vi "main_VI.vi"() -> ()   [LabVIEW 2011]
doc: "This example VI shows how to use thermocouples to take a temperature measurement.\n\nNote:\nFor front panel measurements, make sure the Input switch is in the out position(F)\nFor plug-in card measurements, make sure the Input switch is in the in poisition(R)"
uses:
  <instrlib>/Keithley 622x LV 2009/Configure/Source/Typedefs/KE622x -- Current Level.ctl
  <instrlib>/Keithley 622x LV 2009/Typedefs/KE622x -- On Off Control.ctl
  <vilib>/Utility/file.llb/Write To Spreadsheet File (string).vi
  sub_VIs/west_controller/p6100_write.vi
  <vilib>/addons/Fuzzy Logic/FL Fuzzy Controller (MISO).vi
  <instrlib>/Keithley 27XX/Public/Data/Read Multiple Direct.vi
  sub_VIs/west_controller/p6100_write_setpoint.vi
  <instrlib>/Keithley 27XX/Keithley 27XX.lvlib
  <instrlib>/Keithley 622x LV 2009/Keithley 622x.lvlib
  <vilib>/addons/Fuzzy Logic/NI_Fuzzy_Logic_API.lvlib
panel:
  in  "Current Level (A) In":T1=0.1 min=-0.105 max=0.105 format="%.4p"
  out "Seebeck Graph":cluster{"Y":dbl[], "Y":dbl[]}[](graph)=[{"Y"=[29.390292420231198], "Y"=[134.49214421747814]}]
  out "Resistivity Graph":cluster{"Y":dbl[], "Y":dbl[]}[](graph)=[{"Y"=[29.33802939652643], "Y"=[inf]}]
  out "Temp Graph":cluster{"Y":dbl[], "Y":dbl[]}[](graph)=[{"Y"=[0.0, 0.0, 0.0, 0.0, 0.0, 0.0, 0.0, 0.0, 0.0, 0.0, 0.0, 0.0, 0.0, 0.0, 0.0, 0.0, 0.0, 0.0, 0.0, 0.0, 0.0, 0.0, 0.0, 0.0, 0.0, 0.0, 0.0, 0.0, 0.0, 0.0, 0.0, 0.0, 0.0, 0.0, 0.0, 0.0, 0.0, 0.0, 0.0, 0.0, 0.0, 0.0, 0.0, 0.0, 0.0, 0.0, 0.0, 0.0, 0.0, 0.0, 0.0, 0.0, 0.0, 0.0, 0.0, 0.0, 0.0, 0.0, 0.0, 0.0, 0.0, 0.0, 0.0, 0.0, 0.0, 0.0, 0.0, 0.0, 0.0, 0.0, 0.0, 0.0, 0.0, 0.0, 0.0, 0.0, 0.0, 0.0, 0.0, 0.0, 0.0, 0.0, 0.0, 0.0, 0.0, 0.0, 0.0, 0.0, 0.0, 0.0, 0.0, 0.0, 0.0, 0.0, 0.0, 0.0, 0.0, 0.0, 0.0, 0.0], "Y"=[22.79692727272725, 0.0, 0.0, 0.0, 0.0, 0.0, 0.0, 0.0, 0.0, 0.0, 0.0, 0.0, 0.0, 0.0, 0.0, 0.0, 0.0, 0.0, 0.0, 0.0, 0.0, 0.0, 0.0, 0.0, 0.0, 0.0, 0.0, 0.0, 0.0, 0.0, 0.0, 0.0, 0.0, 0.0, 0.0, 0.0, 0.0, 0.0, 0.0, 0.0, 0.0, 0.0, 0.0, 0.0, 0.0, 0.0, 0.0, 0.0, 0.0, 0.0, 0.0, 0.0, 0.0, 0.0, 0.0, 0.0, 0.0, 0.0, 0.0, 0.0, 0.0, 0.0, 0.0, 0.0, 0.0, 0.0, 0.0, 0.0, 0.0, 0.0, 0.0, 0.0, 0.0, 0.0, 0.0, 0.0, 0.0, 0.0, 0.0, 0.0, 0.0, 0.0, 0.0, 0.0, 0.0, 0.0, 0.0, 0.0, 0.0, 0.0, 0.0, 0.0, 0.0, 0.0, 0.0, 0.0, 0.0, 0.0, 0.0, 0.0]}, {"Y"=[0.0, 0.0, 0.0, 0.0, 0.0, 0.0, 0.0, 0.0, 0.0, 0.0, 0.0, 0.0, 0.0, 0.0, 0.0, 0.0, 0.0, 0.0, 0.0, 0.0, 0.0, 0.0, 0.0, 0.0, 0.0, 0.0, 0.0, 0.0, 0.0, 0.0, 0.0, 0.0, 0.0, 0.0, 0.0, 0.0, 0.0, 0.0, 0.0, 0.0, 0.0, 0.0, 0.0, 0.0, 0.0, 0.0, 0.0, 0.0, 0.0, 0.0, 0.0, 0.0, 0.0, 0.0, 0.0, 0.0, 0.0, 0.0, 0.0, 0.0, 0.0, 0.0, 0.0, 0.0, 0.0, 0.0, 0.0, 0.0, 0.0, 0.0, 0.0, 0.0, 0.0, 0.0, 0.0, 0.0, 0.0, 0.0, 0.0, 0.0, 0.0, 0.0, 0.0, 0.0, 0.0, 0.0, 0.0, 0.0, 0.0, 0.0, 0.0, 0.0, 0.0, 0.0, 0.0, 0.0, 0.0, 0.0, 0.0, 0.0], "Y"=[29.252771602137226, 0.0, 0.0, 0.0, 0.0, 0.0, 0.0, 0.0, 0.0, 0.0, 0.0, 0.0, 0.0, 0.0, 0.0, 0.0, 0.0, 0.0, 0.0, 0.0, 0.0, 0.0, 0.0, 0.0, 0.0, 0.0, 0.0, 0.0, 0.0, 0.0, 0.0, 0.0, 0.0, 0.0, 0.0, 0.0, 0.0, 0.0, 0.0, 0.0, 0.0, 0.0, 0.0, 0.0, 0.0, 0.0, 0.0, 0.0, 0.0, 0.0, 0.0, 0.0, 0.0, 0.0, 0.0, 0.0, 0.0, 0.0, 0.0, 0.0, 0.0, 0.0, 0.0, 0.0, 0.0, 0.0, 0.0, 0.0, 0.0, 0.0, 0.0, 0.0, 0.0, 0.0, 0.0, 0.0, 0.0, 0.0, 0.0, 0.0, 0.0, 0.0, 0.0, 0.0, 0.0, 0.0, 0.0, 0.0, 0.0, 0.0, 0.0, 0.0, 0.0, 0.0, 0.0, 0.0, 0.0, 0.0, 0.0, 0.0]}, {"Y"=[0.0, 0.0, 0.0, 0.0, 0.0, 0.0, 0.0, 0.0, 0.0, 0.0, 0.0, 0.0, 0.0, 0.0, 0.0, 0.0, 0.0, 0.0, 0.0, 0.0, 0.0, 0.0, 0.0, 0.0, 0.0, 0.0, 0.0, 0.0, 0.0, 0.0, 0.0, 0.0, 0.0, 0.0, 0.0, 0.0, 0.0, 0.0, 0.0, 0.0, 0.0, 0.0, 0.0, 0.0, 0.0, 0.0, 0.0, 0.0, 0.0, 0.0, 0.0, 0.0, 0.0, 0.0, 0.0, 0.0, 0.0, 0.0, 0.0, 0.0, 0.0, 0.0, 0.0, 0.0, 0.0, 0.0, 0.0, 0.0, 0.0, 0.0, 0.0, 0.0, 0.0, 0.0, 0.0, 0.0, 0.0, 0.0, 0.0, 0.0, 0.0, 0.0, 0.0, 0.0, 0.0, 0.0, 0.0, 0.0, 0.0, 0.0, 0.0, 0.0, 0.0, 0.0, 0.0, 0.0, 0.0, 0.0, 0.0, 0.0], "Y"=[29.52781323832517, 0.0, 0.0, 0.0, 0.0, 0.0, 0.0, 0.0, 0.0, 0.0, 0.0, 0.0, 0.0, 0.0, 0.0, 0.0, 0.0, 0.0, 0.0, 0.0, 0.0, 0.0, 0.0, 0.0, 0.0, 0.0, 0.0, 0.0, 0.0, 0.0, 0.0, 0.0, 0.0, 0.0, 0.0, 0.0, 0.0, 0.0, 0.0, 0.0, 0.0, 0.0, 0.0, 0.0, 0.0, 0.0, 0.0, 0.0, 0.0, 0.0, 0.0, 0.0, 0.0, 0.0, 0.0, 0.0, 0.0, 0.0, 0.0, 0.0, 0.0, 0.0, 0.0, 0.0, 0.0, 0.0, 0.0, 0.0, 0.0, 0.0, 0.0, 0.0, 0.0, 0.0, 0.0, 0.0, 0.0, 0.0, 0.0, 0.0, 0.0, 0.0, 0.0, 0.0, 0.0, 0.0, 0.0, 0.0, 0.0, 0.0, 0.0, 0.0, 0.0, 0.0, 0.0, 0.0, 0.0, 0.0, 0.0, 0.0]}]
  in  "Comments":string="Esto es una prueba"
  in  "play":bool
  in  "stop":bool
  out "Tab Control 2":enum32{"Page 1", "Page 3"}(tab)
  in  "D (mm)":dbl=7.5
  in  "H (mm)":dbl=1.3
  in  "B (mm)":dbl
  in  "A (mm)":dbl
  in  "L (mm)":dbl
  in  "Select type":u16(ring) items=["Cylinder", "Rectangular"]
  in  "file path":path
  in  "SetPoint Top":dbl
  in  "SetPoint Bottom":dbl
  # "SAMPLE TYPE"
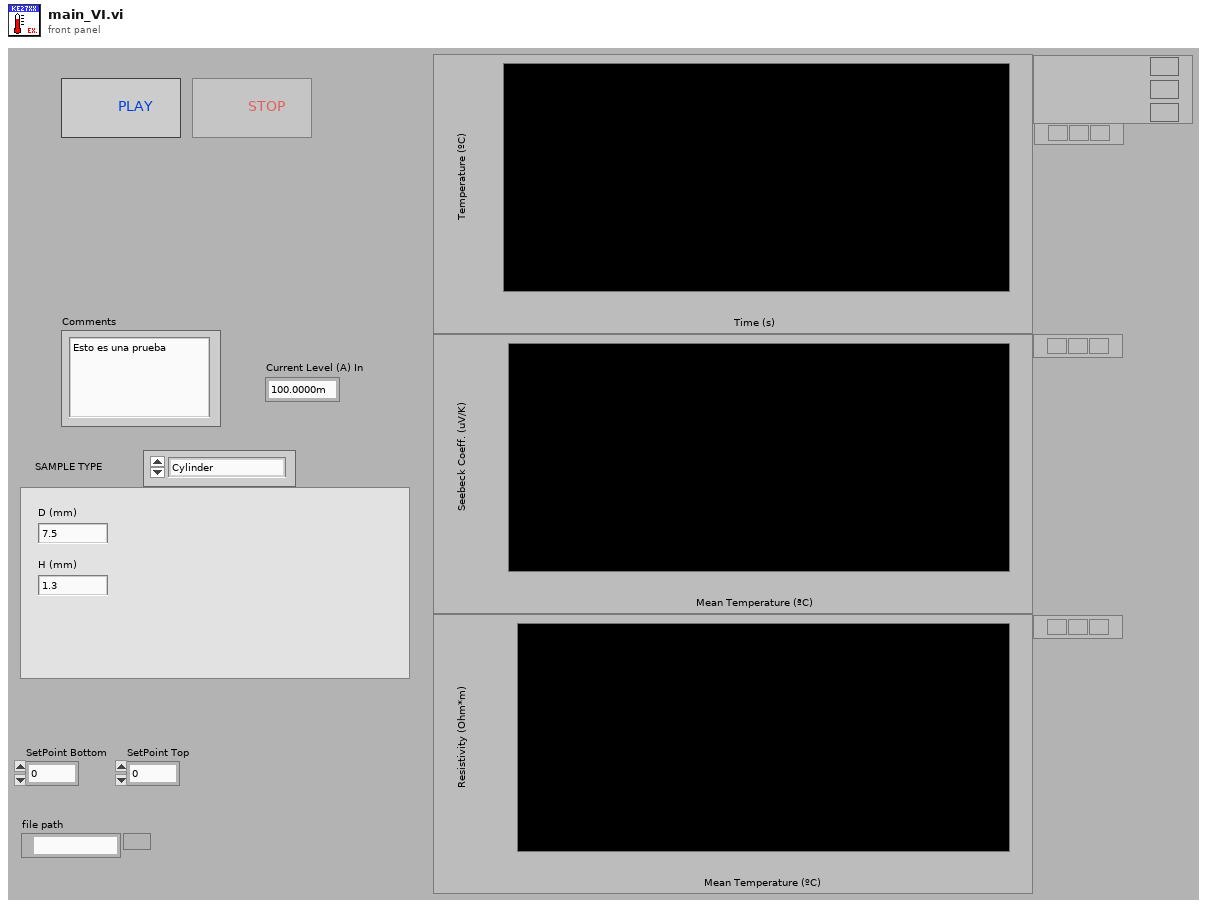
[diagram p1: front panel]
types:
  T1 = typedef "Keithley 622x.lvlib/KE622x -- Current Level.ctl" = dbl
  T2 = cluster{"Baud Rate (9600)":u32, "Flow Control (1: XON/XOFF)":u16, "Termination Char (0:CR)":u16}
  T3 = cluster{"Mode":enum16{"RTU", "ASCII"}, "Slave Bottom":u8, "Slave Top":u8}
  T4 = enum8{"Enabled", "Disabled", "Disabled and Grayed Out"}
  T5 = typedef "NI_Fuzzy_Logic_API.lvlib/FL System.ctl" = cluster{"input variables":T6[], "output variables":T6[], "rules":T9[], "defuzzification method":T15, "description":string, "user MF interpolating polynomials":T16[]}
  T6 = typedef "NI_Fuzzy_Logic_API.lvlib/FL Variable.ctl" = cluster{"name":string, "range":dbl[], "MFs":T7[]}
  T7 = typedef "NI_Fuzzy_Logic_API.lvlib/FL Membership Function.ctl" = cluster{"name":string, "shape":T8, "points":dbl[], "color":u32, "user-defined shape index":i32}
  T8 = typedef "NI_Fuzzy_Logic_API.lvlib/FL Membership Function Shape.ctl" = u16
  T9 = typedef "NI_Fuzzy_Logic_API.lvlib/FL Rule.ctl" = cluster{"antecedents":T10[], "antecedent connective":T12, "consequents":T13[], "consequent implication":T14, "degree of support":dbl}
  T10 = typedef "NI_Fuzzy_Logic_API.lvlib/FL Antecedent.ctl" = cluster{"Var Index":i32, "MF Index":i32, "Cond":T11}
  T11 = typedef "FL Modifier.ctl" = u16
  T12 = typedef "NI_Fuzzy_Logic_API.lvlib/FL Antecedent Connective.ctl" = u16
  T13 = typedef "NI_Fuzzy_Logic_API.lvlib/FL Consequent.ctl" = cluster{"Var Index":i32, "MF Index":i32, "Cond":T11}
  T14 = typedef "NI_Fuzzy_Logic_API.lvlib/FL Consequent Implication.ctl" = u16
  T15 = typedef "NI_Fuzzy_Logic_API.lvlib/FL Defuzzification.ctl" = u16
  T16 = typedef "NI_Fuzzy_Logic_API.lvlib/FL Interpolating polynomials.ctl" = cluster{"X":dbl[], "Y":dbl[], "Y(x) coeff":dbl[][], "X(y) coeff":dbl[][], "Area(y) coeff":dbl[][], "coa_x(y) coeff":dbl[][]}
  T17 = typedef "Keithley 622x.lvlib/KE622x -- On Off Control.ctl" = enum16{"Off", "On"}
  T18 = cluster{"Data Out[0]":dbl, "Data Out[1]":dbl, "Data Out[2]":dbl, "Data Out[3]":dbl, "Data Out[4]":dbl, "Data Out[5]":dbl, "Data Out[6]":dbl, "Data Out[7]":dbl, "Data Out[8]":dbl}
  T19 = cluster{"[0]":dbl, "[1]":dbl, "[2]":dbl, "[3]":dbl, "[4]":dbl, "[5]":dbl, "[6]":dbl, "[7]":dbl, "[8]":dbl}
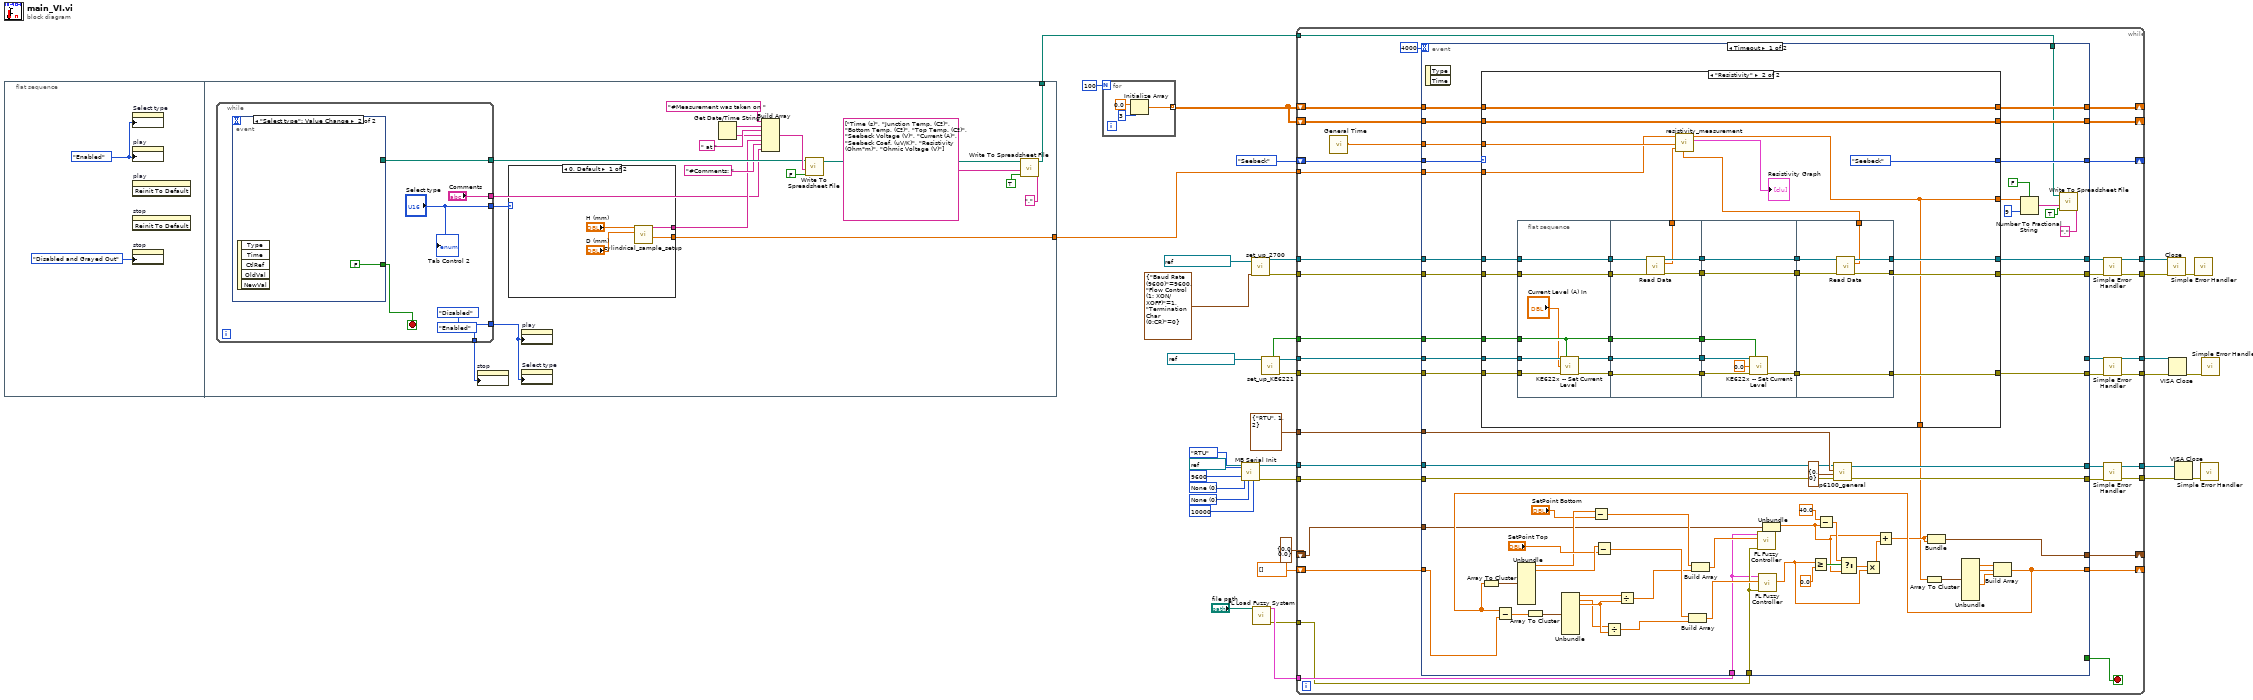
[diagram p0: block diagram]
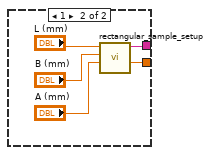
[diagram p2: hidden frame]
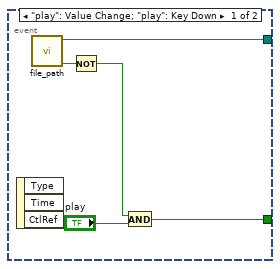
[diagram p3: hidden frame]
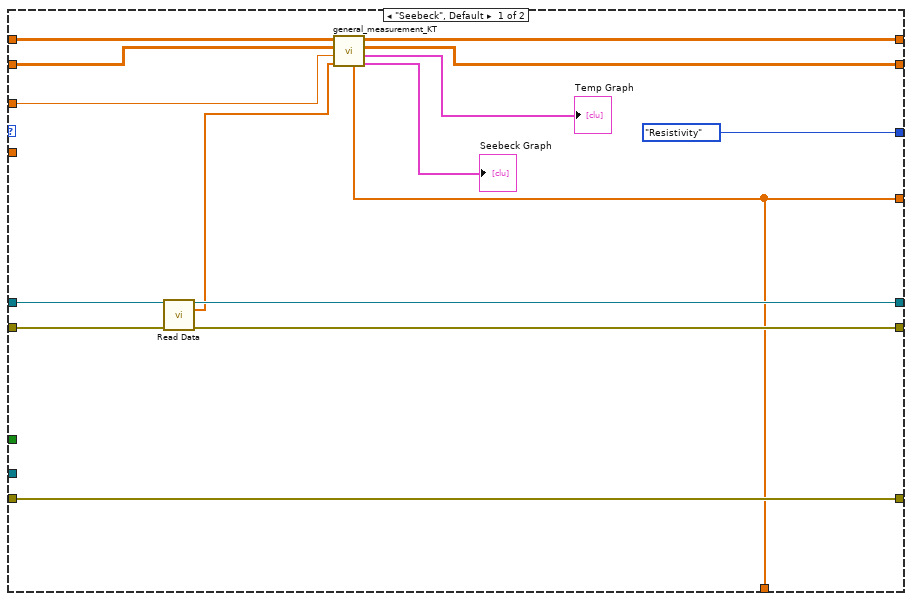
[diagram p4: hidden frame]
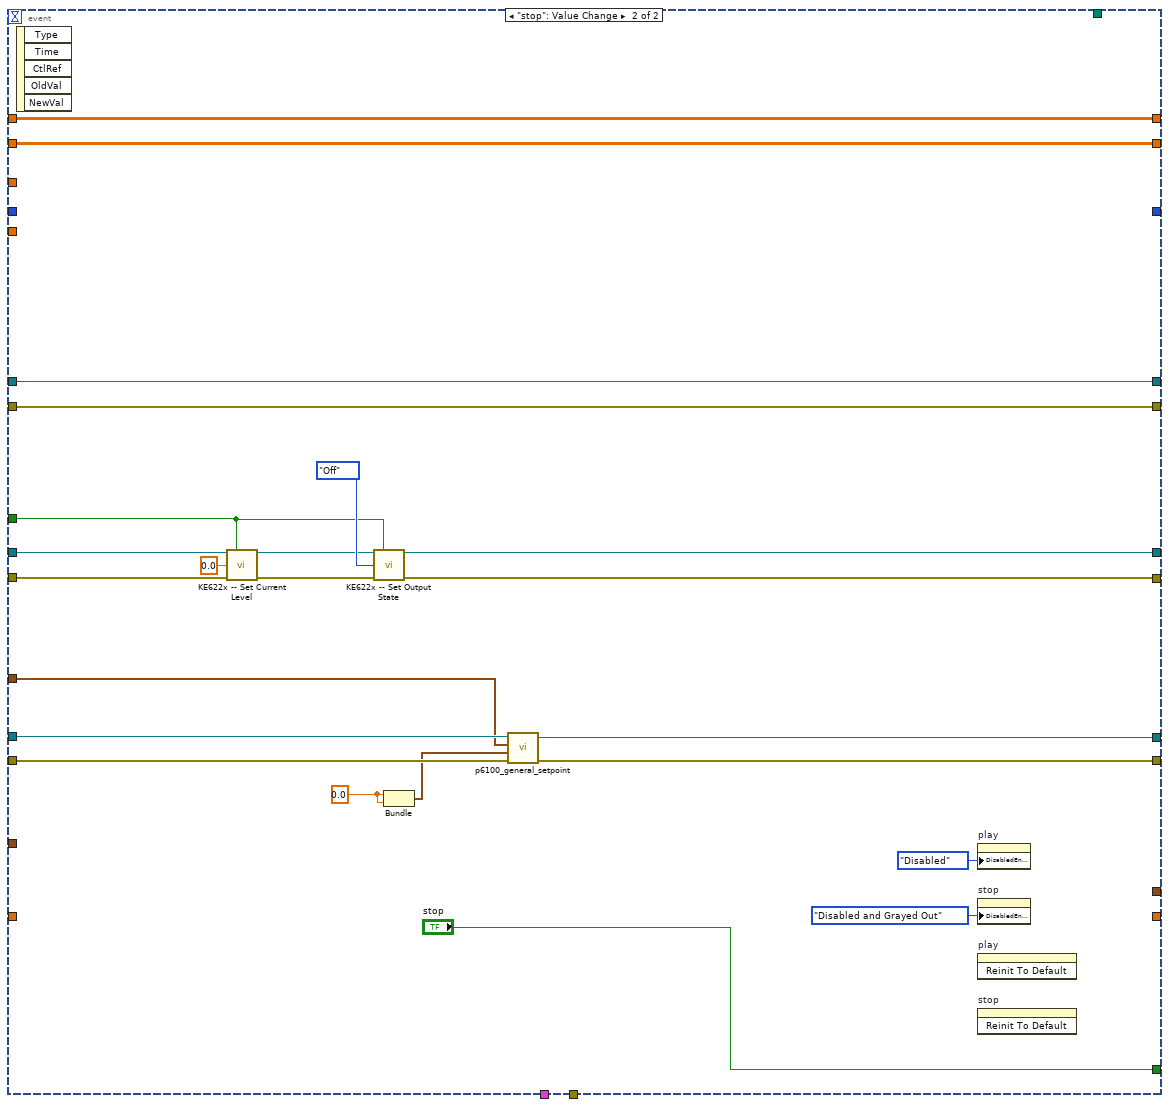
[diagram p5: hidden frame]
diagram:
  w28 = u16 0 items=["None", "XON/XOFF", "RTS/CTS", "XON/XOFF & RTS/CTS", "DTR/DSR", "XON/XOFF & DTR/DSR"] ("Flow Control")
  w29 = u16 0 items=["None", "Odd", "Even", "Mark", "Space"] ("Parity")
  n1 = flat-sequence {
    tunnel: [w42] -> w2
    tunnel: [w47] -> w1
    frame #0 {
      w37 = T4."Enabled" ("Disabled")
      n2 = property on="Select type" class="Ring (strict)"("DisabledEnum"=w37) -> ()  [unwired: 2 in, 2 out]
      n3 = property on="play" class="Bool"("DisabledEnum"=w37) -> ()  [unwired: 2 in, 2 out]
      n4 = invoke on="play" class="Bool" method="Reinit To Default"() -> ()  [unwired: 3 in, 3 out]
      n5 = invoke on="stop" class="Bool" method="Reinit To Default"() -> ()  [unwired: 3 in, 3 out]
      n6 = property on="stop" class="Bool"("DisabledEnum"=T4."Disabled and Grayed Out" ("Disabled")) -> ()  [unwired: 2 in, 2 out]
    }
    frame #1 {
      n7 = while {
        tunnel: [T4."Enabled" ("Disabled")] -> w52
        tunnel: [T4."Disabled" ("Disabled")] -> w39
        tunnel: [w70] -> w51
        tunnel: ["Select type"] -> w41
        tunnel: ["Comments"] -> w40
        stop <- w67 stop-if-true
        n8 = event shown="[1] \"Select type\": Value Change" {
          selector: _ -> [_ _]
          dyn-events: _ -> [_ _]
          timeout: _ -> [_ _]
          tunnel: [w77 _] -> w70
          tunnel: [w73 FALSE] -> w67
          event "play": Value Change; "play": Key Down {
            n9 = event-data() -> ()  [unwired: 1 in, 3 out]
            n10 = call "file_path.vi"() -> ("cancelled"=w76:bool, "selected path"=w77:path)  [unwired: 10 in]
            n11 = Not(x=w76) -> (.not. x?=w75:bool)
            n12 = And(x=w75, y="play") -> (x .and. y?=w73:bool)
          }
          event "Select type": Value Change {
            n13 = event-data() -> ()  [unwired: 1 in, 5 out]
          }
        }
        "Tab Control 2" <- "Select type"
      }
      n14 = property on="stop" class="Bool"("DisabledEnum"=w52) -> ()  [unwired: 2 in, 2 out]
      n15 = case shown="0, Default" w41 {
        tunnel: [w58 w63] -> w42
        tunnel: [w59 w62] -> w43
        frame 0, Default {
          n16 = call "cylindrical_sample_setup.vi"("D (mm)"="D (mm)", "H (mm)"="H (mm)") -> ("Result"=w58:dbl, "spreadsheet string"=w59:string)  [unwired: 8 in]
        }
        frame 1 {
          n17 = call "rectangular_sample_setup.vi"("A (mm)"="A (mm)", "B (mm)"="B (mm)", "L (mm)"="L (mm)") -> ("Result"=w63:dbl, "spreadsheet string"=w62:string)  [unwired: 7 in]
        }
      }
      n18 = property on="play" class="Bool"("DisabledEnum"=w39) -> ()  [unwired: 2 in, 2 out]
      n19 = property on="Select type" class="Ring (strict)"("DisabledEnum"=w39) -> ()  [unwired: 2 in, 2 out]
      n20 = Get Date/Time String() -> (date string=w54:string, time string=w46:string)  [unwired: 3 in]
      n21 = Build Array("#Measurement was taken on ", w54, " at " ("element"), w46, w43, "#Comments: " ("element"), w40) -> (w57:string[])
      n22 = call-poly <vilib>:"Write To Spreadsheet File.vi"("append to file? (new file:F)"=FALSE, "1D data"=w57, "file path (dialog if empty)"=w51) -> ("new file path (Not A Path if cancelled)"=w44:path)  [unwired: 5 in]
      n23 = call-poly <vilib>:"Write To Spreadsheet File.vi"("delimiter (\\t)"="," ("delimiter (\\t)"), "append to file? (new file:F)"=TRUE, "1D data"=string[] ["Time (s)", "Junction Temp. (Cº)", "Bottom Temp. (Cº)", "Top Temp. (Cº)", "Seebeck Voltage (V)", "Current (A)", "Seebeck Coef. (uV/K)", "Resistivity (Ohm*m)", "Ohmic Voltage (V)"] ("Headers"), "file path (dialog if empty)"=w44) -> ("new file path (Not A Path if cancelled)"=w47:path)  [unwired: 4 in]
    }
  }
  n24 = for {
    N: 100 -> [_]
    tunnel: [w81] -> w15 mode=indexing
    n25 = Initialize Array(0.0 ("element"), 3 ("dimension size")) -> (w81:dbl[])
  }
  n26 = call <vilib>:"MB Serial Init.vi"("Timeout"=u32 10000, "Flow Control"=w28, "Mode"=enum16{"RTU", "ASCII"}."RTU", "Parity"=w29, "Baud Rate"=u32 9600, "VISA resource name"=refnum<visa-resource-name> "COM6") -> ("error out"=w24:errorcluster, "VISA resource name out"=w25:refnum<visa-resource-name>)  [unwired: 4 in]
  n27 = call "set_up_2700.vi"("Serial Configuration"=T2 {"Baud Rate (9600)"=9600, "Flow Control (1: XON/XOFF)"=1, "Termination Char (0:CR)"=0}, "VISA Refnum in"=refnum<visa-resource-name> "GPIB0::16::INSTR" ("VISA resource 2700")) -> ("error out"=w35:errorcluster, "VISA Refnum out"=w34:refnum<visa-resource-name>)  [unwired: 8 in]
  n28 = call <vilib>:"FL Load Fuzzy System.vi"("file path"="file path") -> ("error out"=w7:errorcluster, "fuzzy system out"=w8:T5)  [unwired: 9 in]
  n29 = call "set_up_KE6221.vi"("VISA Refnum in"=refnum<visa-resource-name> "GPIB0::12::INSTR" ("VISA resource 6221")) -> ("error out"=w17:errorcluster, "VISA Refnum out"=w18:refnum<visa-resource-name>, "Check For SCPI Errors? (T)"=w5:bool)  [unwired: 8 in]
  n30 = while {
    tunnel: w35 -> [w115]
    tunnel: w34 -> [w114]
    tunnel: [w92] -> w33
    tunnel: [w113] -> w32
    tunnel: w25 -> [w112]
    tunnel: w24 -> [w111]
    tunnel: T3 {"Mode"=enum."RTU", "Slave Bottom"=1, "Slave Top"=2} ("Serial Parameters") -> [w110]
    tunnel: [w97] -> w21
    tunnel: [w98] -> w20
    shift-right: [w107] -> _
    shift-left: w15 -> [w91]
    shift-right: [w108] -> _
    shift-left: w15 -> [w109]
    tunnel: w18 -> [w105]
    tunnel: w17 -> [w104]
    tunnel: w5 -> [w103]
    tunnel: [w94] -> w13
    shift-right: [w100] -> _
    shift-left: enum16{"Seebeck", "Resistivity"}."Seebeck" -> [w101]
    tunnel: [w96] -> w11
    shift-right: [w88] -> _
    shift-left: dbl[] [] ("Data Out") -> [w90]
    tunnel: w8 -> [w87]
    tunnel: w7 -> [w86]
    shift-right: [w85] -> _
    shift-left: cluster{"output value":dbl, "output value":dbl} {"output value"=0.0, "output value"=0.0} ("upper limit") -> [w84]
    tunnel: w1 -> [w83]
    tunnel: w2 -> [w82]
    stop <- w102 stop-if-true
    n31 = call "General Time"() -> ("Elapsed Time (s)"=w89:dbl)  [unwired: 12 in, 7 out]
    n32 = event shown="[0] Timeout" {
      selector: _ -> [_ _]
      dyn-events: _ -> [_ _]
      timeout: 4000 -> [_ _]
      tunnel: w115 -> [w175 w268]
      tunnel: w114 -> [w176 w269]
      tunnel: [w180 w268] -> w93
      tunnel: [w179 w269] -> w113
      tunnel: w112 -> [w140 w276]
      tunnel: w111 -> [w139 w273]
      tunnel: w110 -> [w141 w272]
      tunnel: [w143 w275] -> w97
      tunnel: [w142 w274] -> w99
      tunnel: [_ "stop"] -> w102
      tunnel: w91 -> [w173 w266]
      tunnel: w109 -> [w174 w267]
      tunnel: [w178 w267] -> w108
      tunnel: [w177 w266] -> w107
      tunnel: w105 -> [w170 w262]
      tunnel: w104 -> [w172 w265]
      tunnel: w103 -> [w169 w260]
      tunnel: [w171 w259] -> w95
      tunnel: w101 -> [w168 _]
      tunnel: [w167 _] -> w100
      tunnel: [_ w258] -> w96
      tunnel: w90 -> [w149 _]
      tunnel: w89 -> [w166 _]
      tunnel: [w144 _] -> w88
      tunnel: w87 -> [w150 _]
      tunnel: w86 -> [w151 _]
      tunnel: [w125 _] -> w85
      tunnel: w84 -> [w136 _]
      tunnel: w83 -> [w119 _]
      tunnel: w82 -> [w117 _]
      event Timeout {
        n33 = event-data() -> ()  [unwired: 1 in, 2 out]
        n34 = case shown="\"Resistivity\"" w168 {
          tunnel: [w195 w214] -> w180
          tunnel: [w194 w219] -> w179
          tunnel: [w193 w225] -> w178
          tunnel: [w192 w224] -> w177
          tunnel: w176 -> [w191 w223]
          tunnel: w175 -> [w190 w217]
          tunnel: w174 -> [w189 w225]
          tunnel: w173 -> [w188 w224]
          tunnel: w172 -> [w185 w209]
          tunnel: [w185 w206] -> w171
          tunnel: w170 -> [_ w212]
          tunnel: w169 -> [_ w205]
          tunnel: w166 -> [w182 w201]
          tunnel: [enum16{"Seebeck", "Resistivity"}."Resistivity" enum16{"Seebeck", "Resistivity"}."Seebeck"] -> w167
          tunnel: [w181 w197] -> w123
          tunnel: [w181 w197] -> w121
          tunnel: w117 -> [_ w196]
          frame "Seebeck", Default {
            n35 = call-poly <instrlib>:"Read Data.vi"("VISA resource name"=w191, "error in (no error)"=w190) -> ("VISA resource name out"=w194:refnum<visa-resource-name>, "Measurement Data"=w183:dbl[], "error out"=w195:errorcluster)  [unwired: 8 in, 3 out]
            n36 = call "general_measurement_KT.vi"("Data Keithley"=w183, "General Time"=w182, "Array Time In"=w188, "Array Temp In"=w189) -> ("Seebeck Graph"=→"Seebeck Graph":cluster{"Y":dbl[], "Y":dbl[]}[], "Temp Graph"=→"Temp Graph":cluster{"Y":dbl[], "Y":dbl[]}[], "Array Time Out"=w192:dbl[][], "Array Temp Out"=w193:dbl[][], "Data Out"=w181:dbl[])  [unwired: 3 in]
          }
          frame "Resistivity" {
            n37 = flat-sequence {
              tunnel: w223 -> [w233]
              tunnel: [w233] -> w222
              tunnel: [w232] -> w218
              tunnel: w217 -> [w232]
              tunnel: [w230] -> w213
              tunnel: w212 -> [w231]
              tunnel: [w228] -> w210
              tunnel: w209 -> [w229]
              tunnel: w205 -> [w227]
              tunnel: [w227] -> w203
              tunnel: w222 -> [w241]
              tunnel: [w240] -> w221
              tunnel: w218 -> [w239]
              tunnel: [w238] -> w215
              tunnel: w213 -> [w237]
              tunnel: [w237] -> w211
              tunnel: w210 -> [w236]
              tunnel: [w236] -> w208
              tunnel: [w235] -> w204
              tunnel: w203 -> [w235]
              tunnel: [w234] -> w200
              tunnel: w221 -> [w248]
              tunnel: [w248] -> w220
              tunnel: [w247] -> w216
              tunnel: w215 -> [w247]
              tunnel: w211 -> [w246]
              tunnel: w208 -> [w245]
              tunnel: [w244] -> w207
              tunnel: w204 -> [w243]
              tunnel: w220 -> [w254]
              tunnel: [w253] -> w219
              tunnel: w216 -> [w252]
              tunnel: [w251] -> w214
              tunnel: w207 -> [w250]
              tunnel: [w250] -> w206
              tunnel: [w249] -> w199
              frame #0 {
                n38 = call <instrlib>:"KE622x -- Set Current Level.vi"("Resource In"=w231, "Check For SCPI Errors? (T)"=w227, "Current Level (A) In"="Current Level (A) In", "error in (no error)"=w229) -> ("Resource Out (dupl)"=w230:refnum<visa-resource-name>, "error out"=w228:errorcluster)  [unwired: 9 in, 1 out]
              }
              frame #1 {
                n39 = call-poly <instrlib>:"Read Data.vi"("VISA resource name"=w241, "error in (no error)"=w239) -> ("VISA resource name out"=w240:refnum<visa-resource-name>, "Measurement Data"=w234:dbl[], "error out"=w238:errorcluster)  [unwired: 8 in, 3 out]
              }
              frame #2 {
                n40 = call <instrlib>:"KE622x -- Set Current Level.vi"("Resource In"=w246, "Check For SCPI Errors? (T)"=w243, "Current Level (A) In"=T1 0.0, "error in (no error)"=w245) -> ("error out"=w244:errorcluster)  [unwired: 9 in, 2 out]
              }
              frame #3 {
                n41 = call-poly <instrlib>:"Read Data.vi"("VISA resource name"=w254, "error in (no error)"=w252) -> ("VISA resource name out"=w253:refnum<visa-resource-name>, "Measurement Data"=w249:dbl[], "error out"=w251:errorcluster)  [unwired: 8 in, 3 out]
              }
            }
            n42 = call "resistivity_measurement.vi"("S-l Ratio"=w196, "General Time"=w201, "Measurement Data 1"=w200, "Measurement Data 2"=w199) -> ("Data Out"=w197:dbl[], "Resistivity Graph"=→"Resistivity Graph":cluster{"Y":dbl[], "Y":dbl[]}[])  [unwired: 3 in]
          }
        }
        n43 = Unbundle(w136) -> ("output value"=w128:dbl)  [unwired: 1 out]
        n44 = Subtract(x=40.0, y=w128) -> (x-y=w132:dbl)
        n45 = call-poly "p6100_general.vi"("VISA in"=w140, "Serial Parameters"=w141, "Setpoint"=cluster{u8, u8} {0, 0}, "error in"=w139) -> ("VISA out"=w143:refnum<visa-resource-name>, "error out"=w142:errorcluster)  [unwired: 1 in, 1 out]
        n46 = Array To Cluster(array=w123) -> (cluster=w165:T18)
        n47 = Unbundle(w165) -> ("Data Out[1]"=w164:dbl, "Data Out[2]"=w163:dbl, "Data Out[5]"=w162:dbl)  [unwired: 6 out]
        n48 = Build Array(w164, w163, w162) -> (w144:dbl[])
        n49 = Array To Cluster(array=w144) -> (cluster=w159:T19)
        n50 = Subtract(x=w144, y=w149) -> (x-y=w152:dbl[])
        n51 = Unbundle(w159) -> ("[0]"=w146:dbl, "[1]"=w148:dbl)  [unwired: 7 out]
        n52 = Array To Cluster(array=w152) -> (cluster=w153:T19)
        n53 = Unbundle(w153) -> ("[0]"=w154:dbl, "[1]"=w155:dbl, "[2]"=w156:dbl)  [unwired: 6 out]
        n54 = Subtract(x=w146, y="SetPoint Bottom") -> (x-y=w160:dbl)
        n55 = Subtract(x=w148, y="SetPoint Top") -> (x-y=w161:dbl)
        n56 = Divide(x=w155, y=w156) -> (x/y=w137:dbl)
        n57 = Divide(x=w154, y=w156) -> (x/y=w138:dbl)
        n58 = Build Array(w161, w137) -> (w158:dbl[])
        n59 = Build Array(w160, w138) -> (w157:dbl[])
        n60 = call-poly <vilib>:"FL Fuzzy Controller.vi"("error in (no error)"=w151, "input values"=w157, "fuzzy system in"=w150) -> ()  [unwired: 4 in, 5 out]
        n61 = call-poly <vilib>:"FL Fuzzy Controller.vi"("error in (no error)"=w151, "input values"=w158, "fuzzy system in"=w150) -> ("output value"=w130:dbl)  [unwired: 4 in, 4 out]
        n62 = Greater Or Equal?(x=w130, y=0.0) -> (x >= y?=w134:bool)
        n63 = Select(t=w132, s=w134, f=w128) -> (s? t:f=w131:dbl)
        n64 = Multiply(x=w131, y=w130) -> (x*y=w129:dbl)
        n65 = Add(x=w128, y=w129) -> (x+y=w126:dbl)
        n66 = Bundle(w126, w126) -> (w125:cluster{dbl, dbl})  [unwired: 1 in]
        n67 = Number To Fractional String(use system decimal point (T)=FALSE, number=w121, precision (6)=i16 9) -> (F-format string=w120:string[])  [unwired: 1 in]
        n68 = call-poly <vilib>:"Write To Spreadsheet File.vi"("delimiter (\\t)"="," ("delimiter (\\t)"), "append to file? (new file:F)"=TRUE, "1D data"=w120, "file path (dialog if empty)"=w119) -> ()  [unwired: 4 in, 1 out]
      }
      event "stop": Value Change {
        w270 = 0.0
        n69 = event-data() -> ()  [unwired: 1 in, 5 out]
        n70 = call <instrlib>:"KE622x -- Set Current Level.vi"("Resource In"=w262, "Check For SCPI Errors? (T)"=w260, "Current Level (A) In"=T1 0.0, "error in (no error)"=w265) -> ("Resource Out (dupl)"=w261:refnum<visa-resource-name>, "error out"=w264:errorcluster)  [unwired: 9 in, 1 out]
        n71 = call <instrlib>:"KE622x -- Set Output State.vi"("Resource In"=w261, "Check For SCPI Errors? (T)"=w260, "Output State"=KE622x_--_On_Off_Control."Off", "error in (no error)"=w264) -> ("Resource Out (dupl)"=w258:refnum<visa-resource-name>, "error out"=w259:errorcluster)  [unwired: 10 in]
        n72 = Bundle(w270, w270) -> (w271:cluster{dbl, dbl})  [unwired: 1 in]
        n73 = call-poly "p6100_general_setpoint.vi"("VISA in"=w276, "Serial Parameters"=w272, "Setpoint"=w271, "error in"=w273) -> ("VISA out"=w275:refnum<visa-resource-name>, "error out"=w274:errorcluster)  [unwired: 1 in, 1 out]
        n74 = property on="play" class="Bool"("DisabledEnum"=T4."Disabled" ("Disabled")) -> ()  [unwired: 2 in, 2 out]
        n75 = property on="stop" class="Bool"("DisabledEnum"=T4."Disabled and Grayed Out" ("Disabled")) -> ()  [unwired: 2 in, 2 out]
        n76 = invoke on="play" class="Bool" method="Reinit To Default"() -> ()  [unwired: 3 in, 3 out]
        n77 = invoke on="stop" class="Bool" method="Reinit To Default"() -> ()  [unwired: 3 in, 3 out]
      }
    }
    n78 = call <vilib>:"Simple Error Handler.vi"("error in (no error)"=w93) -> ("error out"=w92:errorcluster)  [unwired: 1 in, 7 out]
    n79 = call <vilib>:"Simple Error Handler.vi"("error in (no error)"=w95) -> ("error out"=w94:errorcluster)  [unwired: 1 in, 7 out]
    n80 = call <vilib>:"Simple Error Handler.vi"("error in (no error)"=w99) -> ("error out"=w98:errorcluster)  [unwired: 1 in, 7 out]
  }
  n81 = call <instrlib>:"Close.vi"("VISA resource name"=w32, "error in (no error)"=w33) -> ("error out"=w36:errorcluster)  [unwired: 13 in]
  n82 = VISA Close(VISA resource name=w11, error in (no error)=w13) -> (error out=w12:errorcluster)
  n83 = VISA Close(VISA resource name=w21, error in (no error)=w20) -> (error out=w22:errorcluster)
  n84 = call <vilib>:"Simple Error Handler.vi"("error in (no error)"=w36) -> ()  [unwired: 4 in, 5 out]
  n85 = call <vilib>:"Simple Error Handler.vi"("error in (no error)"=w22) -> ()  [unwired: 1 in, 8 out]
  n86 = call <vilib>:"Simple Error Handler.vi"("error in (no error)"=w12) -> ()  [unwired: 4 in, 5 out]
